vi "Set Routing Channel Description.vi"(8 "error in":errorcluster, 10 "description":string, 11 "routing channel in":T1 format="%.0x") -> (0 "error out":errorcluster, 3 "routing channel out":T1 format="%.0x")   [LabVIEW 2020, in "Routing and Faulting Scripting.lvlib"]
doc: "Sets the description for the routing channel."
uses:
  Routing and Faulting Scripting.lvlib
  <vilib>/NI VeriStand/Custom Device API/Custom Device Item Ref.ctl
  <vilib>/NI VeriStand/Custom Device API/Custom Device API.lvlib
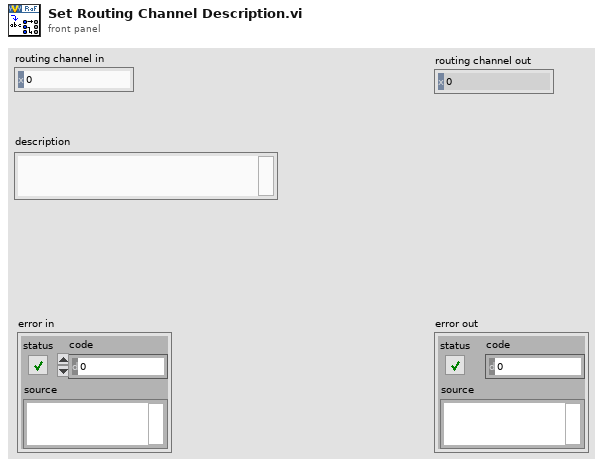
[diagram p1: front panel]
types:
  T1 = typedef "Custom Device API.lvlib/Custom Device Item Ref.ctl" = u64
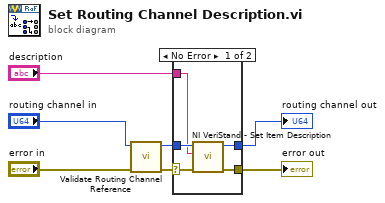
[diagram p0: block diagram]
diagram:
  n1 = call "Validate Routing Channel Reference.vi"("error in"="error in", "routing channel in"="routing channel in") -> ("error out"=w3:errorcluster, "routing channel out"=w1:T1)  [unwired: 8 in]
  n2 = case shown="No Error" w3 {
    selector: w3 -> [w8 w14]
    tunnel: [w10 w14] -> w4
    tunnel: [w11 w13] -> w5
    tunnel: w1 -> [w12 w13]
    tunnel: "description" -> [w9 _]
    frame No Error {
      n3 = call <vilib>:"NI VeriStand - Set Item Description.vi"("error in (no error)"=w8, "Description"=w9, "Item Ref in"=w12) -> ("error out"=w10:errorcluster, "Item Ref out"=w11:T1)  [unwired: 6 in, 1 out]
    }
    frame Error {
    }
  }
  "error out" <- w4
  "routing channel out" <- w5
